vi "FindAngle.vi"(11 "Array in":i32[][](array[numeric])) -> (3 "Angle":dbl format="%0.2f")   [LabVIEW 2017]
uses:
  <vilib>/Analysis/baseanly.llb/Mean (DBL).vi
  <vilib>/Analysis/NI_AALBase.lvlib
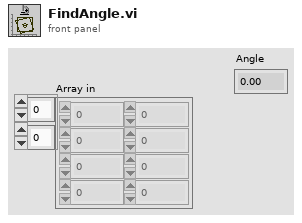
[diagram p1: front panel]
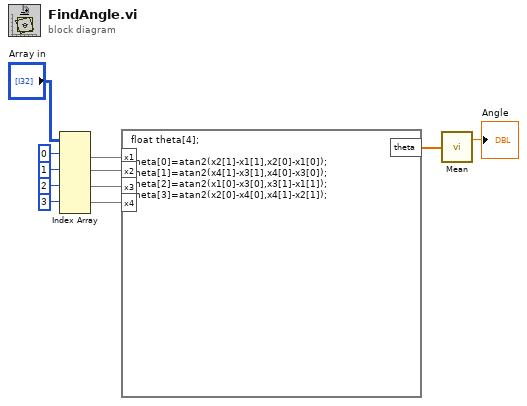
[diagram p0: block diagram]
diagram:
  n1 = Index Array(array="Array in", index (row) #1=0 ("index (row)"), index (row) #2=1 ("index (row)"), index (row) #3=2 ("index (row)"), index (row) #4=3 ("index (row)")) -> (element #1=w8:i32[], element #2=w9:i32[], element #3=w10:i32[], element #4=w11:i32[])  [unwired: 4 in]
  n2 = formula code="float theta[4];\n\ntheta[0]=atan2(x2[1]-x1[1],x2[0]-x1[0]);\ntheta[1]=atan2(x4[1]-x3[1],x4[0]-x3[0]);\ntheta[2]=atan2(x1[0]-x3[0],x3[1]-x1[1]);\ntheta[3]=atan2(x2[0]-x4[0],x4[1]-x2[1]);"("x1"=w8, "x2"=w9, "x3"=w10, "x4"=w11) -> ("theta"=w2:dbl[])
  n3 = call-poly <vilib>:"Mean.vi"("X"=w2) -> ("mean"=→"Angle":dbl)  [unwired: 1 out]
